vi "Poll Epics Variables.vi"(8 "error in (no error)":errorcluster, 10 "Epics Initial Configuration":T1, 11 "Queue in":refnum<queue>) -> (0 "error out":errorcluster)   [LabVIEW 2014]
uses:
  Message Queue/Message Cluster.ctl
  controls/EPICS Configuration.ctl
  Message Queue/Message Queue.lvlib
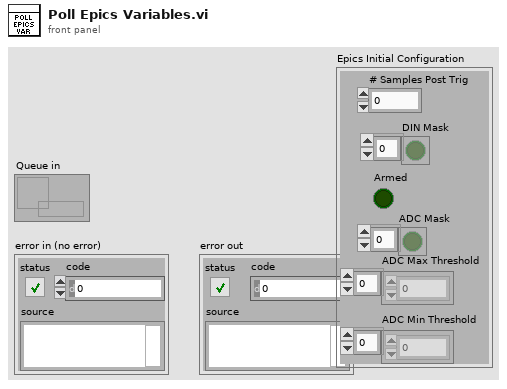
[diagram p1: front panel]
types:
  T1 = typedef "EPICS Configuration.ctl" = cluster{"DIN Mask":bool[], "# Samples Post Trig":u32, "Armed":bool, "ADC Mask":bool[], "ADC Max Threshold":dbl[], "ADC Min Threshold":dbl[]}
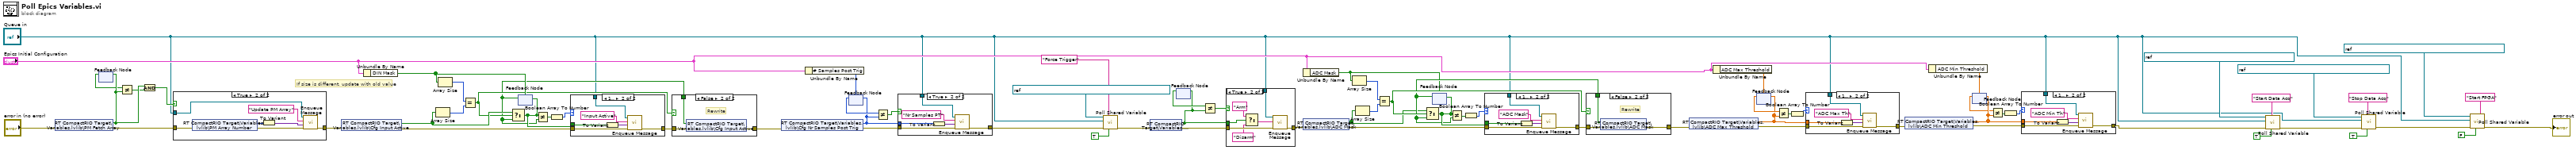
[diagram p0: block diagram]
diagram:
  # "If size is different, update with old value"
  n1 = shared-variable "RT CompactRIO Target\\Variables.lvlib\\PM Fetch Array"(error in="error in (no error)") -> (w74:bool, error out=w72:errorcluster)
  n2 = feedback #1() -> (w73:bool)  [unwired: 1 in]
  n3 = feedback-in #1(w74) -> ()
  n4 = Not Equal?(x=w73, y=w74) -> (x != y?=w70:bool)
  n5 = And(x=w74, y=w70) -> (x .and. y?=w71:bool)
  n6 = case shown="True" w71 {
    tunnel: "Queue in" -> [_ w79]
    tunnel: w72 -> [w75 w82]
    tunnel: [w75 w80] -> w65
    frame False {
    }
    frame True {
      n7 = shared-variable "RT CompactRIO Target\\Variables.lvlib\\PM Array Number"(error in=w82) -> (w77:u8, error out=w81:errorcluster)
      n8 = To Variant(anything=w77) -> (Variant=w76:variant)
      n9 = call "Enqueue Message.vi"("error in (no error)"=w81, "Message Data"=w76, "Message"="Update PM Array", "Message Queue"=w79) -> ("error out"=w80:errorcluster)  [unwired: 6 in, 1 out]
    }
  }
  n10 = shared-variable "RT CompactRIO Target\\Variables.lvlib\\Cfg Input Active"(error in=w65) -> (w57:bool[], error out=w63:errorcluster)
  n11 = Unbundle By Name("Epics Initial Configuration") -> ("DIN Mask"=w62:bool[])
  n12 = Array Size(array=w57) -> (size(s)=w60:i32)
  n13 = Array Size(array=w62) -> (size(s)=w61:i32)
  n14 = Equal?(x=w61, y=w60) -> (x = y?=w54:bool)
  n15 = feedback #2(w62) -> (w52:bool[])
  n16 = Select(t=w57, s=w54, f=w52) -> (s? t:f=w53:bool[])
  n17 = feedback-in #2(w53) -> ()
  n18 = Not Equal?(x=w53, y=w52) -> (x != y?=w59:bool[])
  n19 = Boolean Array To Number(Boolean array=w59) -> (number=w58:u32)
  n20 = case shown="1.." w58 {
    tunnel: w63 -> [w83 w89]
    tunnel: [w83 w88] -> w56
    tunnel: "Queue in" -> [_ w87]
    tunnel: w53 -> [_ w85]
    frame 0, Default {
    }
    frame 1.. {
      n21 = To Variant(anything=w85) -> (Variant=w86:variant)
      n22 = call "Enqueue Message.vi"("error in (no error)"=w89, "Message Data"=w86, "Message"="Input Active", "Message Queue"=w87) -> ("error out"=w88:errorcluster)  [unwired: 6 in, 1 out]
    }
  }
  n23 = case shown="False" w54 {
    tunnel: w56 -> [w90 w93]
    tunnel: [w90 w92] -> w55
    tunnel: w52 -> [_ w91]
    frame True {
    }
    frame False {
      # "Rewrite"
      n24 = shared-variable "RT CompactRIO Target\\Variables.lvlib\\Cfg Input Active"(w91, error in=w93) -> (error out=w92:errorcluster)
    }
  }
  n25 = shared-variable "RT CompactRIO Target\\Variables.lvlib\\Cfg Nr Samples Post Trig"(error in=w55) -> (w46:u32, error out=w48:errorcluster)
  n26 = Unbundle By Name("Epics Initial Configuration") -> ("# Samples Post Trig"=w50:u32)
  n27 = feedback #3(w50) -> (w51:u32)
  n28 = feedback-in #3(w46) -> ()
  n29 = Not Equal?(x=w51, y=w46) -> (x != y?=w49:bool)
  n30 = case shown="True" w49 {
    tunnel: w48 -> [w94 w100]
    tunnel: [w94 w99] -> w47
    tunnel: "Queue in" -> [_ w98]
    tunnel: w46 -> [_ w96]
    frame False {
    }
    frame True {
      n31 = To Variant(anything=w96) -> (Variant=w97:variant)
      n32 = call "Enqueue Message.vi"("error in (no error)"=w100, "Message Data"=w97, "Message"="Nr Samples PT", "Message Queue"=w98) -> ("error out"=w99:errorcluster)  [unwired: 6 in, 1 out]
    }
  }
  n33 = call "Poll Shared Variable.vi"("Reset?"=TRUE, "Message"="Force Trigger", "error in (no error)"=w47, "Message handler"="Queue in", "Refnum in"=refnum<k21> "ni.var.psp://RT CompactRIO Target/Variables/Force Trigger" ("shared variable refnum in")) -> ("error out"=w64:errorcluster)  [unwired: 6 in]
  n34 = shared-variable "RT CompactRIO Target\\Variables.lvlib\\Arm"(error in=w64) -> (w42:bool, error out=w44:errorcluster)
  n35 = feedback #4() -> (w45:bool)  [unwired: 1 in]
  n36 = feedback-in #4(w42) -> ()
  n37 = Not Equal?(x=w45, y=w42) -> (x != y?=w43:bool)
  n38 = case shown="True" w43 {
    tunnel: [w101 w107] -> w33
    tunnel: w44 -> [w101 w108]
    tunnel: "Queue in" -> [_ w106]
    tunnel: w42 -> [_ w105]
    frame False {
    }
    frame True {
      n39 = Select(t="Arm", s=w105, f="Disarm") -> (s? t:f=w102:string)
      n40 = call "Enqueue Message.vi"("error in (no error)"=w108, "Message"=w102, "Message Queue"=w106) -> ("error out"=w107:errorcluster)  [unwired: 7 in, 1 out]
    }
  }
  n41 = shared-variable "RT CompactRIO Target\\Variables.lvlib\\ADC Mask"(error in=w33) -> (w31:bool[], error out=w32:errorcluster)
  n42 = Unbundle By Name("Epics Initial Configuration") -> ("ADC Mask"=w30:bool[])
  n43 = Array Size(array=w30) -> (size(s)=w41:i32)
  n44 = Array Size(array=w31) -> (size(s)=w40:i32)
  n45 = Equal?(x=w41, y=w40) -> (x = y?=w36:bool)
  n46 = feedback #5(w30) -> (w34:bool[])
  n47 = Select(t=w31, s=w36, f=w34) -> (s? t:f=w35:bool[])
  n48 = feedback-in #5(w35) -> ()
  n49 = Not Equal?(x=w35, y=w34) -> (x != y?=w39:bool[])
  n50 = Boolean Array To Number(Boolean array=w39) -> (number=w38:u32)
  n51 = case shown="1.." w38 {
    tunnel: w32 -> [w109 w115]
    tunnel: [w109 w114] -> w37
    tunnel: "Queue in" -> [_ w113]
    tunnel: w35 -> [_ w111]
    frame 0, Default {
    }
    frame 1.. {
      n52 = To Variant(anything=w111) -> (Variant=w112:variant)
      n53 = call "Enqueue Message.vi"("error in (no error)"=w115, "Message Data"=w112, "Message"="ADC Mask", "Message Queue"=w113) -> ("error out"=w114:errorcluster)  [unwired: 6 in, 1 out]
    }
  }
  n54 = case shown="False" w36 {
    tunnel: w37 -> [w116 w119]
    tunnel: [w116 w118] -> w25
    tunnel: w34 -> [_ w117]
    frame True {
    }
    frame False {
      # "Rewrite"
      n55 = shared-variable "RT CompactRIO Target\\Variables.lvlib\\ADC Mask"(w117, error in=w119) -> (error out=w118:errorcluster)
    }
  }
  n56 = shared-variable "RT CompactRIO Target\\Variables.lvlib\\ADC Max Threshold"(error in=w25) -> (w26:dbl[], error out=w27:errorcluster)
  n57 = Unbundle By Name("Epics Initial Configuration") -> ("ADC Max Threshold"=w28:dbl[])
  n58 = feedback #6(w28) -> (w29:dbl[])
  n59 = feedback-in #6(w26) -> ()
  n60 = Not Equal?(x=w29, y=w26) -> (x != y?=w17:bool[])
  n61 = Boolean Array To Number(Boolean array=w17) -> (number=w18:u32)
  n62 = case shown="1.." w18 {
    tunnel: w27 -> [w120 w126]
    tunnel: [w120 w125] -> w19
    tunnel: "Queue in" -> [_ w124]
    tunnel: w26 -> [_ w122]
    frame 0, Default {
    }
    frame 1.. {
      n63 = To Variant(anything=w122) -> (Variant=w123:variant)
      n64 = call "Enqueue Message.vi"("error in (no error)"=w126, "Message Data"=w123, "Message"="ADC Max Th", "Message Queue"=w124) -> ("error out"=w125:errorcluster)  [unwired: 6 in, 1 out]
    }
  }
  n65 = shared-variable "RT CompactRIO Target\\Variables.lvlib\\ADC Min Threshold"(error in=w19) -> (w24:dbl[], error out=w23:errorcluster)
  n66 = Unbundle By Name("Epics Initial Configuration") -> ("ADC Min Threshold"=w22:dbl[])
  n67 = feedback #7(w22) -> (w21:dbl[])
  n68 = feedback-in #7(w24) -> ()
  n69 = Not Equal?(x=w21, y=w24) -> (x != y?=w14:bool[])
  n70 = Boolean Array To Number(Boolean array=w14) -> (number=w15:u32)
  n71 = case shown="1.." w15 {
    tunnel: w23 -> [w127 w133]
    tunnel: [w127 w132] -> w20
    tunnel: "Queue in" -> [_ w131]
    tunnel: w24 -> [_ w129]
    frame 0, Default {
    }
    frame 1.. {
      n72 = To Variant(anything=w129) -> (Variant=w130:variant)
      n73 = call "Enqueue Message.vi"("error in (no error)"=w133, "Message Data"=w130, "Message"="ADC Min Th", "Message Queue"=w131) -> ("error out"=w132:errorcluster)  [unwired: 6 in, 1 out]
    }
  }
  n74 = call "Poll Shared Variable.vi"("Reset?"=TRUE, "Message"="Start Data Acq", "error in (no error)"=w20, "Message handler"="Queue in", "Refnum in"=refnum<k21> "ni.var.psp://RT CompactRIO Target/Variables/PM Set on" ("shared variable refnum in")) -> ("error out"=w7:errorcluster)  [unwired: 6 in]
  n75 = call "Poll Shared Variable.vi"("Reset?"=TRUE, "Message"="Stop Data Acq", "error in (no error)"=w7, "Message handler"="Queue in", "Refnum in"=refnum<k21> "ni.var.psp://RT CompactRIO Target/Variables/PM Set Off" ("shared variable refnum in")) -> ("error out"=w3:errorcluster)  [unwired: 6 in]
  n76 = call "Poll Shared Variable.vi"("Reset?"=FALSE, "Message"="Start FPGA", "error in (no error)"=w3, "Message handler"="Queue in", "Refnum in"=refnum<k21> "ni.var.psp://RT CompactRIO Target/Variables/Reset Interlock" ("shared variable refnum in")) -> ("error out"=→"error out":errorcluster)  [unwired: 6 in]
